vi "Queue Driver.vi"(0 "States":string[](array[string]), 2 "Name":string, 11 "Error in":errorcluster, 13 "Operation":T1) -> (4 "Dequeued State":string, 15 "Error out":errorcluster)   [LabVIEW 2020]
doc: "This VI is used as LV2 queue for states in state machine"
uses:
  Typedefs/Queue operations.ctl
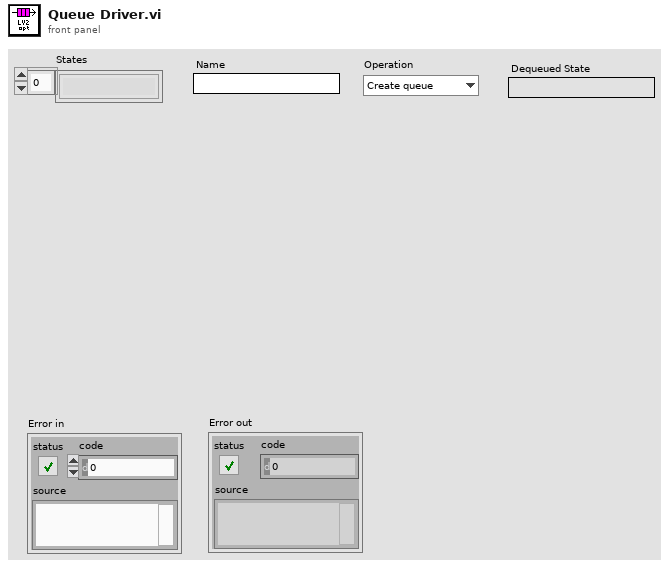
[diagram p1: front panel]
types:
  T1 = typedef "Queue operations.ctl" = enum16{"Create queue", "Enqueue", "Enstack", "Dequeue", "Flush queue", "Release queue"}
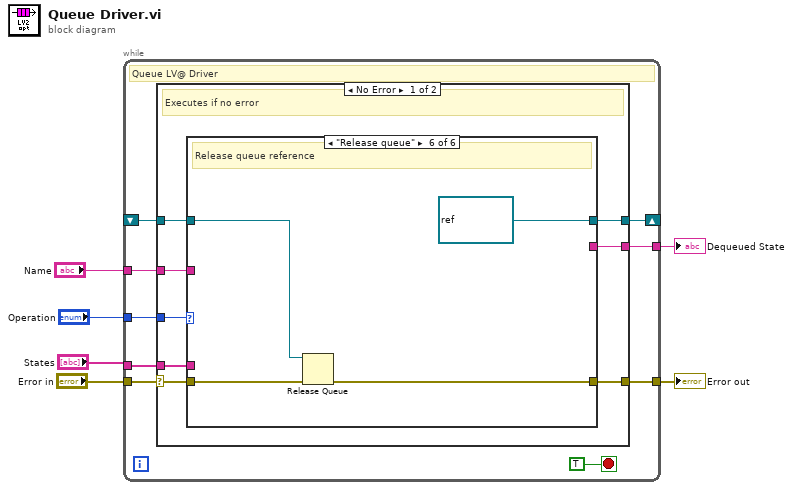
[diagram p0: block diagram]
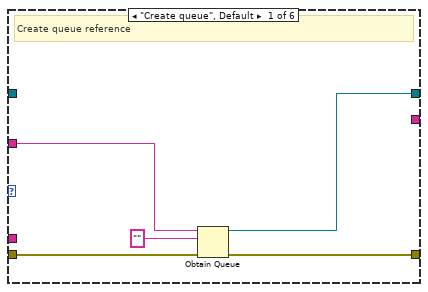
[diagram p2: hidden frame]
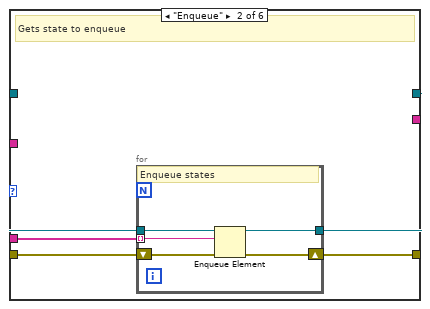
[diagram p3: hidden frame]
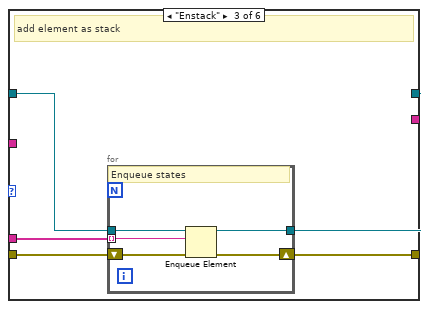
[diagram p4: hidden frame]
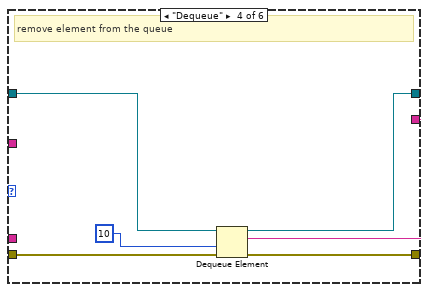
[diagram p5: hidden frame]
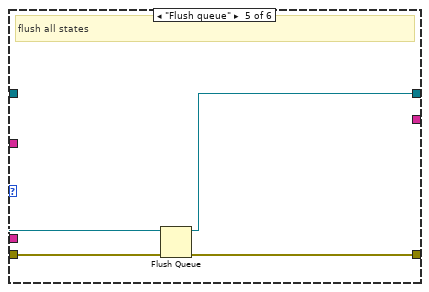
[diagram p6: hidden frame]
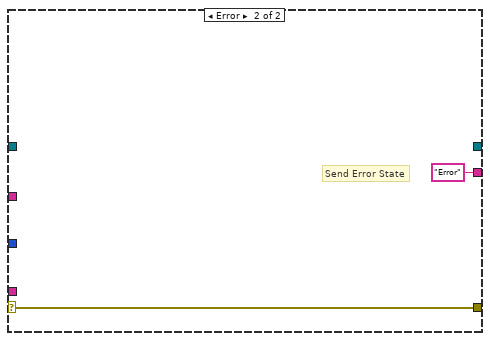
[diagram p7: hidden frame]
diagram:
  n1 = while {
    tunnel: "Error in" -> [w15]
    tunnel: [w14] -> w5
    tunnel: "Operation" -> [w13]
    tunnel: "Name" -> [w12]
    shift-right: [w11] -> _
    shift-left: _ -> [w9]
    tunnel: "States" -> [w10]
    tunnel: [w8] -> w1
    stop <- TRUE stop-if-true
    # "Queue LV@ Driver"
    n2 = case shown="No Error" w15 {
      selector: w15 -> [w21 w64]
      tunnel: [w20 w64] -> w14
      tunnel: w13 -> [w23 _]
      tunnel: w12 -> [w22 _]
      tunnel: [w19 _] -> w11
      tunnel: w10 -> [w18 _]
      tunnel: w9 -> [w17 _]
      tunnel: [w16 "Error"] -> w8
      frame No Error {
        # "Executes if no error"
        n3 = case shown="\"Release queue\"" w23 {
          tunnel: w22 -> [w26 _ _ _ _ _]
          tunnel: w21 -> [w28 w31 w43 w54 w58 w62]
          tunnel: [w27 w29 w42 w53 w57 w61] -> w20
          tunnel: [w24 w30 w39 w51 w55 refnum<queue> refnum ("queue out")] -> w19
          tunnel: w18 -> [_ w33 w41 _ _ _]
          tunnel: w17 -> [_ w32 w40 w52 w56 w60]
          tunnel: [_ _ _ w49 _ _] -> w16
          frame "Create queue", Default {
            # "Create queue reference"
            n4 = Obtain Queue(name (unnamed)=w26, element data type="", error in (no error)=w28) -> (queue out=w24:refnum<queue>, error out=w27:errorcluster)  [unwired: 2 in, 1 out]
          }
          frame "Enqueue" {
            # "Gets state to enqueue"
            n5 = for {
              tunnel: w32 -> [w36]
              tunnel: [w35] -> w30
              tunnel: w33 -> [w34] mode=indexing
              shift-right: [w38] -> w29
              shift-left: w31 -> [w37]
              # "Enqueue states"
              n6 = Enqueue Element(queue=w36, element=w34, error in (no error)=w37) -> (queue out=w35:refnum<queue>, error out=w38:errorcluster)  [unwired: 1 in, 1 out]
            }
          }
          frame "Enstack" {
            # "add element as stack"
            n7 = for {
              tunnel: w40 -> [w46]
              tunnel: [w45] -> w39
              tunnel: w41 -> [w44] mode=indexing
              shift-right: [w48] -> w42
              shift-left: w43 -> [w47]
              # "Enqueue states"
              n8 = Enqueue Element(queue=w46, element=w44, error in (no error)=w47) -> (queue out=w45:refnum<queue>, error out=w48:errorcluster)  [unwired: 1 in, 1 out]
            }
          }
          frame "Dequeue" {
            # "remove element from the queue"
            n9 = Dequeue Element(queue=w52, timeout in ms (-1)=10, error in (no error)=w54) -> (queue out=w51:refnum<queue>, element=w49:string, error out=w53:errorcluster)  [unwired: 1 out]
          }
          frame "Flush queue" {
            # "flush all states"
            n10 = Flush Queue(queue=w56, error in (no error)=w58) -> (queue out=w55:refnum<queue>, error out=w57:errorcluster)  [unwired: 1 out]
          }
          frame "Release queue" {
            # "Release queue reference"
            n11 = Release Queue(queue=w60, error in (no error)=w62) -> (error out=w61:errorcluster)  [unwired: 1 in, 2 out]
          }
        }
      }
      frame Error {
        # "Send Error State"
      }
    }
  }
  "Error out" <- w5
  "Dequeued State" <- w1
